vi "createInboundChannel.vi"(8 "error in (no error)":errorcluster, 11 "Connection in":refnum<class "Connection.lvclass">) -> (0 "error out":errorcluster, 2 "Authorization":T1, 3 "Connection out":refnum<class "Connection.lvclass">)   [LabVIEW 2013, in "Connection_GOSPL.lvlib" / "Connection.lvclass"]
uses:
  Connection.lvclass
  auth -- cluster.ctl
  Connection.lvclass/Connection.ctl
  <vilib>/LabVIEW Open Source Project/Unicity/RandomStringGenerator/RandomStringGenerator.lvclass
  Store/Store.lvclass
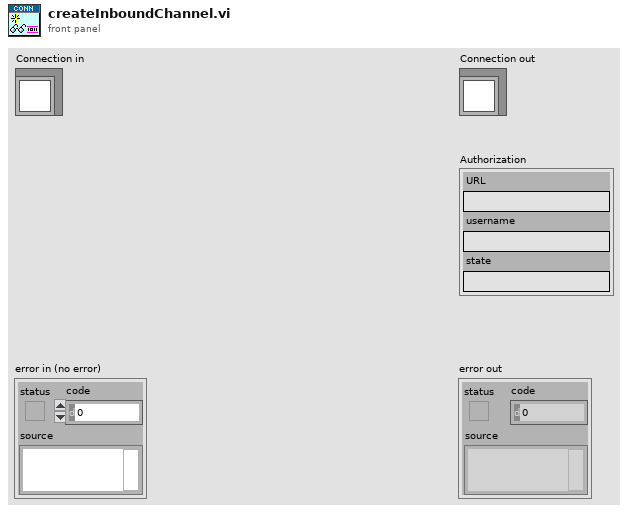
[diagram p1: front panel]
types:
  T1 = typedef "Connection_GOSPL.lvlib/Connection.lvclass/auth -- cluster.ctl" = cluster{"URL":string, "username":string, "state":string}
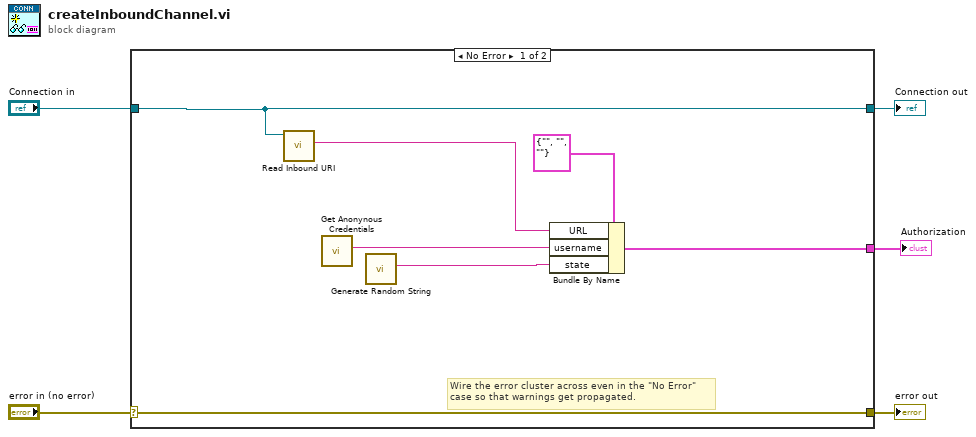
[diagram p0: block diagram]
diagram:
  n1 = case shown="No Error" "error in (no error)" {
    selector: "error in (no error)" -> [w12 w14]
    tunnel: [w12 w14] -> w4
    tunnel: [w7 w13] -> w2
    tunnel: "Connection in" -> [w7 w13]
    tunnel: [w10 _] -> w1
    frame No Error {
      # "Wire the error cluster across even in the \"No Error\"\ncase so that warnings get propagated."
      n2 = call "Read Inbound URI.vi"("Connection in"=w7) -> ("Inbound URI"=w6:string)  [unwired: 9 in, 1 out]
      n3 = call "Get Anonynous Credentials.vi"() -> ("Anonymous username"=w8:string)  [unwired: 10 in, 1 out]
      n4 = call <vilib>:"Generate Random String.vi"() -> ("Random String"=w11:string)  [unwired: 11 in]
      n5 = Bundle By Name(cluster=T1 {"URL"="", "username"="", "state"=""} ("Authorization"), "URL"=w6, "username"=w8, "state"=w11) -> (w10:T1)
    }
    frame Error {
    }
  }
  "error out" <- w4
  "Connection out" <- w2
  "Authorization" <- w1
